vi "MatrixSwitchSingle.vi"(7 "Switch action":u16(ring) items=["Open", "Close"], 8 "error in (no error)":errorcluster, 9 "Matrix Y":i32=1 min=1 max=12 step=1, 10 "Matrix X":i32=1 min=1 max=12 step=1, 11 "LXIPXISwitching in":refnum<class "LXIPXISwitching.lvclass">) -> (0 "error out":errorcluster, 2 "command string":string, 3 "LXIPXISwitching out":refnum<class "LXIPXISwitching.lvclass">)   [LabVIEW 2018, in "LXIPXISwitching.lvclass"]
uses:
  LXIPXISwitching.lvclass
  LXIPXISwitching.lvclass/LXIPXISwitching.ctl
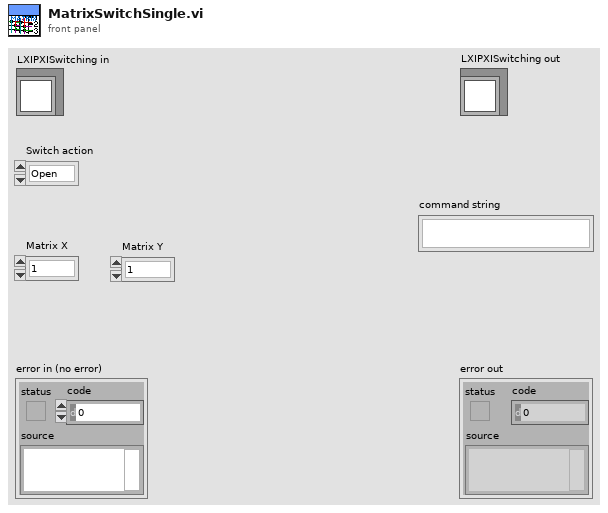
[diagram p1: front panel]
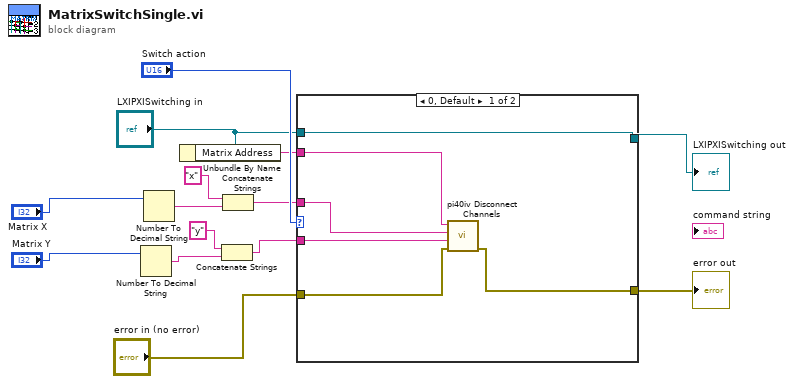
[diagram p0: block diagram]
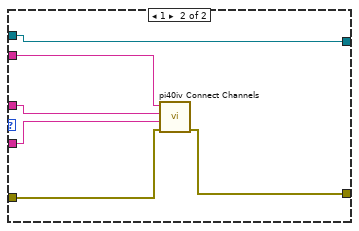
[diagram p2: hidden frame]
diagram:
  n1 = Number To Decimal String(number="Matrix Y") -> (decimal integer string=w8:string)  [unwired: 1 in]
  n2 = Number To Decimal String(number="Matrix X") -> (decimal integer string=w10:string)  [unwired: 1 in]
  n3 = Unbundle By Name("LXIPXISwitching in") -> ("Matrix Address"=w5:string)
  n4 = Concatenate Strings("y" ("string"), w8) -> (w7:string)
  n5 = Concatenate Strings("x" ("string"), w10) -> (w6:string)
  n6 = case shown="0, Default" "Switch action" {
    tunnel: w7 -> [w20 w25]
    tunnel: w6 -> [w19 w26]
    tunnel: w5 -> [w18 w24]
    tunnel: "error in (no error)" -> [w17 w23]
    tunnel: [w16 w22] -> w3
    tunnel: [w15 w21] -> w1
    tunnel: "LXIPXISwitching in" -> [w15 w21]
    frame 0, Default {
      n7 = call <instrlib>:"pi40iv Disconnect Channels.vi"("error in (no error)"=w17, "channel 2"=w20, "channel 1"=w19, "instrument handle"=w18) -> ("error out"=w16:errorcluster)  [unwired: 6 in, 1 out]
    }
    frame 1 {
      n8 = call <instrlib>:"pi40iv Connect Channels.vi"("error in (no error)"=w23, "channel 2"=w25, "channel 1"=w26, "instrument handle"=w24) -> ("error out"=w22:errorcluster)  [unwired: 6 in, 1 out]
    }
  }
  "error out" <- w3
  "LXIPXISwitching out" <- w1
